vi "writeToFile.vi"(8 "error in (no error)":errorcluster, 10 "New Record String":string, 11 "Handler.File.Text in":refnum<class "Handler.File.Text.lvclass">) -> (0 "error out":errorcluster, 3 "Handler.File.Text out":refnum<class "Handler.File.Text.lvclass">)   [LabVIEW 2017, in "Error Log.lvlib" / "Handler.File.Text.lvclass"]
uses:
  Handler.File.Text.lvclass
  Handler.File.Text.lvclass/Handler.File.Text.ctl
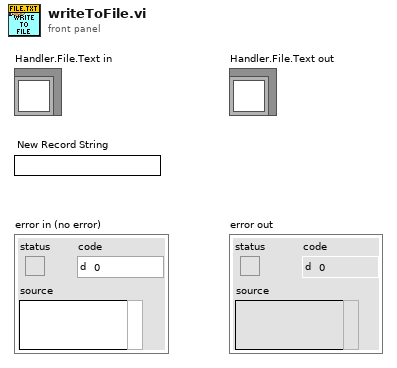
[diagram p1: front panel]
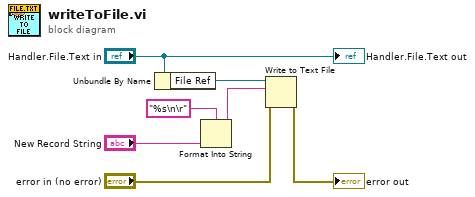
[diagram p0: block diagram]
diagram:
  n1 = Unbundle By Name("Handler.File.Text in") -> ("File Ref"=w6:refnum<file>)
  n2 = Format Into String(format string="%s\n\r", "New Record String") -> (resulting string=w2:string)  [unwired: 2 in, 1 out]
  n3 = Write to Text File(file (use dialog)=w6, text=w2, error in="error in (no error)") -> (error out=→"error out":errorcluster)  [unwired: 1 in, 2 out]
  "Handler.File.Text out" <- "Handler.File.Text in"
